vi "SDI Multi-Axis Simultaneous Start.vi"() -> ()   [LabVIEW 2014]
uses:
  <vilib>/Platform/TimedLoop/XDataNode/timing_clust.ctl
  <vilib>/Platform/TimedLoop/XDataNode/nitl_modes.ctl
  <vilib>/Platform/TimedLoop/XDataNode/wakeup.ctl
  <vilib>/Motion/plugins/PluginFramework/nismSDIFramework.SetFrameworkMode.multi.vi
  <vilib>/Motion/Express/_s/nimc.ex.clearFaults.clearFaults.axis.vi
  <vilib>/Motion/Express/_s/nimc.ex.power.power.axis.vi
  <vilib>/Motion/Express/_s/nimc.ex.read.readExecutionData.axis.vi
  <vilib>/Motion/Express/_s/nimc.ex.stopMove.stop.axis.modeDecelerate.vi
  <vilib>/Motion/Express/_s/nimc.ex.straightLineMove.startStraightLineMove.axis.modeRelative.0.vi
  <vilib>/Motion/BlockNode/FB.NIMotion.xnode
  <vilib>/Platform/TimedLoop/XDataNode/XDataNode.xnode
  <vilib>/Platform/TimedLoop/XDataNode/XDNodeRunTimeDep.lvlib
  <vilib>/Motion/plugins/SDI Plug-in - Delta ASDA/Template SoftMotion Drive Interface Plug-in Class.lvclass
panel:
  out "Move Done":bool
  out "Move Position":cluster{dbl, dbl}(graph)
  in  "Axis 2":refnum<k21>="Axis 2"
  in  "Velocity 2":dbl=3000.0
  in  "Position 2":dbl=7000.0
  in  "Stop Move":bool
  out "error out":errorcluster
  in  "Velocity 1":dbl=1000.0
  in  "Position 1":dbl=-4000.0
  out "Example Done":bool
  in  "Axis 1":refnum<k21>="Axis 1"
  # "Move Constraints"
  # "Notes: \n1. This example uses preconfigured settings that may not be appropriate for your motion system. Review and update the axis settings using the Axis Configuration dialog box. Right-click each axis and select Properties to open the Axis Configuration dialog box. \n2. Running this example automatically activates all axes. Disable the \"Enable Drive on Transition to Active Mode\" option on the General Settings page of the Axis Configuration dialog box to prevent axes from activating when the VI runs.\n3. This example uses the default smoothing input to automatically calculate deceleration and jerk values. To specify these move constraints, connect a control to the \"smoothing\" input to adjust the value to your requirements. \n\nFor information about using this example in an actual motion system, refer to ni.com/info and enter Info Code nismex."
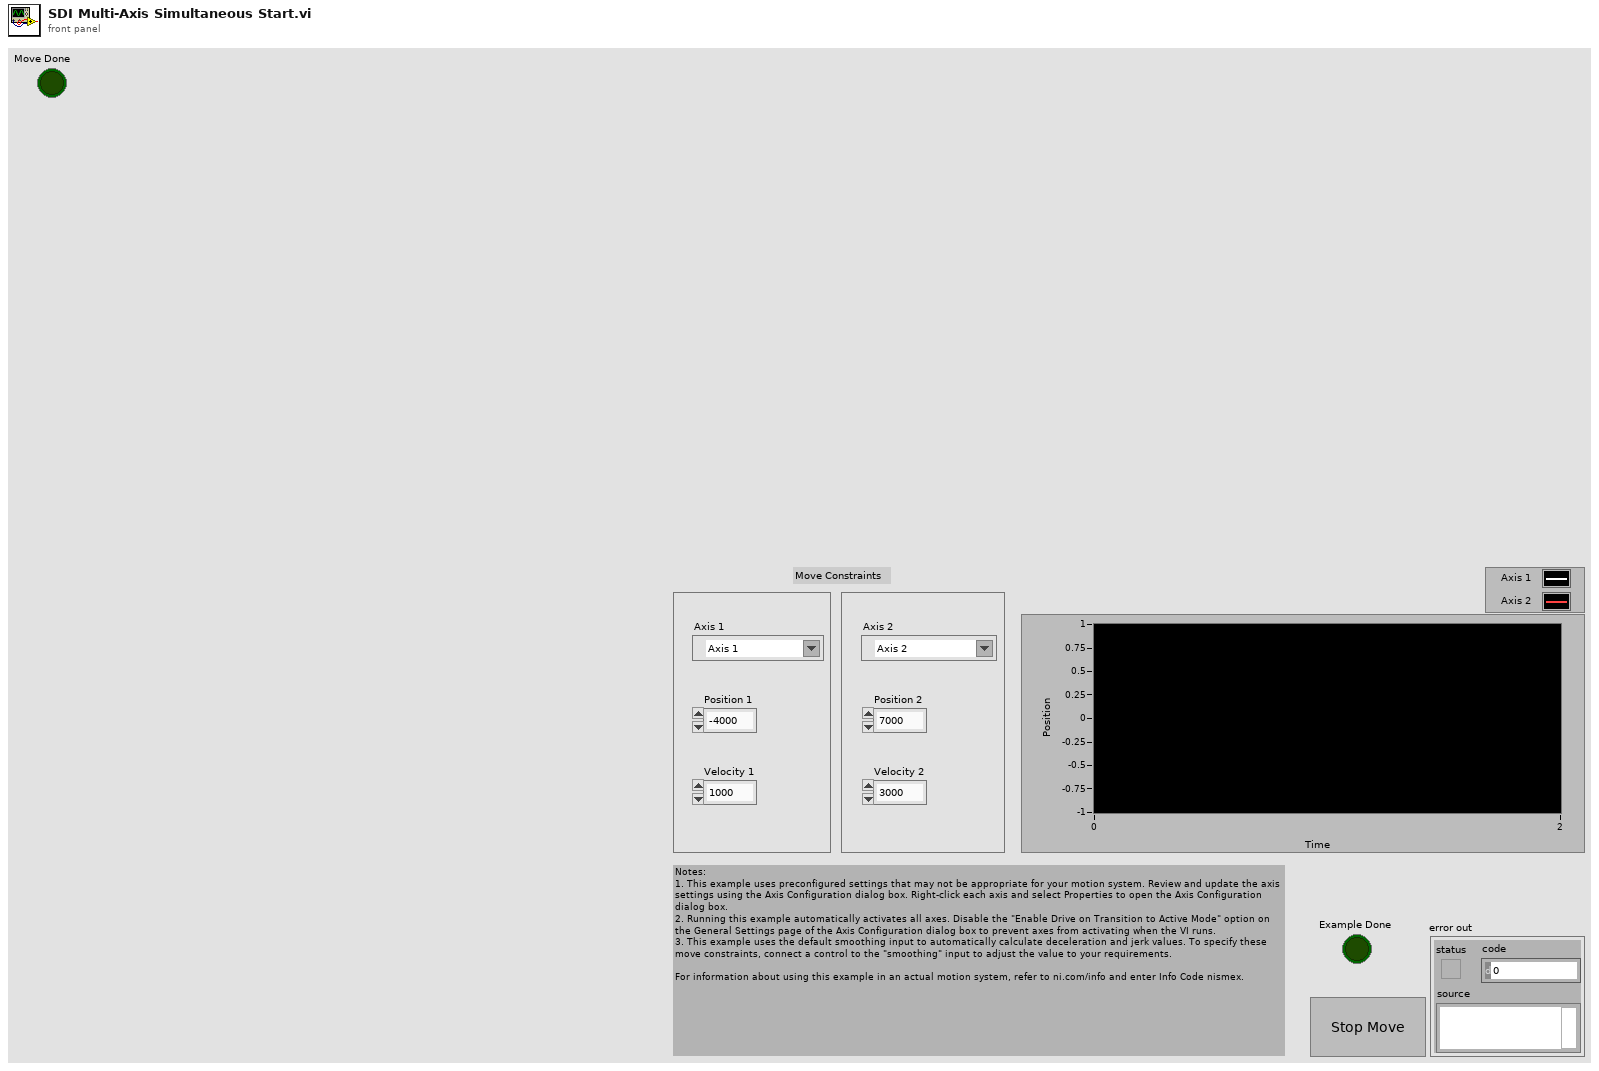
[diagram p1: front panel]
types:
  T1 = typedef "XDNodeRunTimeDep.lvlib/timing_clust.ctl" = cluster{"Expected End [f-1]":u64, "Actual End [f-1]":u64, "Finished Late? [f-1]":bool, "Expected End [i-1]":u64, "Actual End [i-1]":u64, "Finished Late? [i-1]":bool, "Expected Start [i]":u64, "Actual Start [i]":u64, "Expected Start [f]":u64, "Actual Start [f]":u64, "Source Name":string, "Structure Name":string, "Period":i64, "Deadline":i64, "Offset":i64, "Start":i64, "Priority":i32, "Timeout":i32, "Mode":T2, "Wakeup Reason":T3, "Error":errorcluster, "Source Type":string, "Secondary Source Type":string, "Global End Time":u64, "Global Start Time":u64, "Frame Duration":u64, "Iteration Duration":u64, "Assigned CPU":i32, "I/O Scan Engine Mode":u32}
  T2 = typedef "XDNodeRunTimeDep.lvlib/nitl_modes.ctl" = enum32{"No Change", "Process missed periods, maintain original phase", "Discard missed periods, maintain original phase", "Process missed periods, ignore original phase", "Discard missed periods, ignore original phase"}
  T3 = typedef "XDNodeRunTimeDep.lvlib/wakeup.ctl" = enum32{"Normal", "Aborted", "Asynchronous wakeup", "Timing source error", "Timed loop error", "Timeout"}
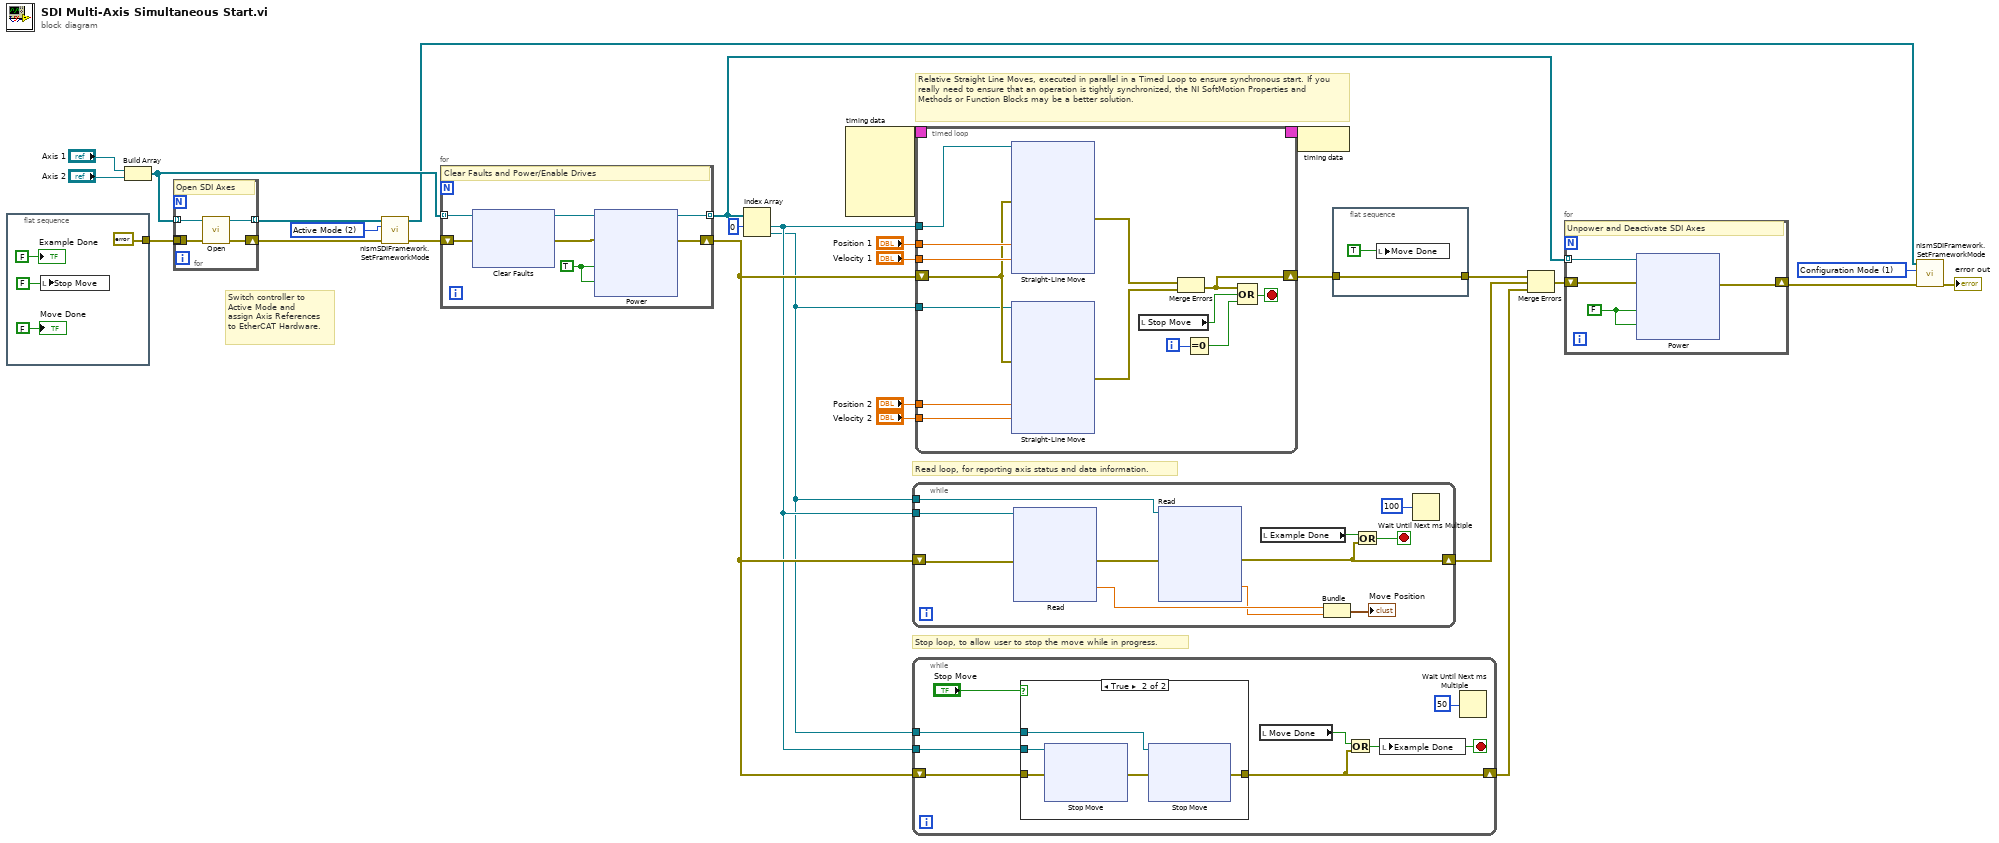
[diagram p0: block diagram]
diagram:
  w8 = 1 items=["Configuration Mode"=1, "Active Mode"=2] ("mode (Active Mode)")
  w18 = 2 items=["Configuration Mode"=1, "Active Mode"=2] ("mode (Active Mode)")
  # "Switch controller to\nActive Mode and \nassign Axis References\nto EtherCAT Hardware."
  # "Relative Straight Line Moves, executed in parallel in a Timed Loop to ensure synchronous start. If you really need to ensure that an operation is tightly synchronized, the NI SoftMotion Properties and Methods or Function Blocks may be a better solution."
  # "Read loop, for reporting axis status and data information."
  # "Stop loop, to allow user to stop the move while in progress."
  n1 = flat-sequence {
    tunnel: [w29] -> _
    tunnel: [w29] -> w11
    frame #0 {
      w29 = errorcluster {"status"=FALSE, "code"=0, "source"=""} ("Error")
      n2 = local write "Stop Move"(FALSE ("Example Done")) -> ()
      "Example Done" <- FALSE ("Example Done")
      "Move Done" <- FALSE ("Example Done")
    }
  }
  n3 = Build Array("Axis 1", "Axis 2") -> (w16:refnum<k21>[])
  n4 = for {
    tunnel: w16 -> [w36] mode=indexing
    tunnel: [w35] -> w15 mode=indexing
    shift-right: [w34] -> w14
    shift-left: _ -> [w33]
    tunnel: w11 -> [_]
    # "Open SDI Axes"
    n5 = call <vilib>:"Open.vi"("error in (no error)"=w33, "Axis"=w36) -> ("error out"=w34:errorcluster, "Base Axis Out"=w35:refnum<class "nismPluginAxisBaseClass.lvclass">)  [unwired: 8 in]
  }
  n6 = call-poly <vilib>:"nismSDIFramework.SetFrameworkMode.vi"("error in (no error)"=w14, "mode (Active Mode)"=w18, "Base Axis In"=w15) -> ("error out"=w17:errorcluster, "Base Axis Out"=w1:refnum<class "nismPluginAxisBaseClass.lvclass">[])  [unwired: 7 in]
  n7 = for {
    tunnel: w16 -> [w39] mode=indexing
    tunnel: [w38] -> w4 mode=indexing
    shift-right: [w41] -> w9
    shift-left: w17 -> [w40]
    w43 = TRUE ("enable axis")
    # "Clear Faults and Power/Enable Drives"
    n8 = xnode ("Clear Faults")("resource"=w39, "error in"=w40) -> ("resource out"=w37:refnum<k21>, "error out"=w42:errorcluster)
    n9 = xnode ("Power")("enable axis"=w43, "enable drive"=w43, "resource"=w37, "error in"=w42) -> ("resource out"=w38:refnum<k21>, "error out"=w41:errorcluster)
  }
  n10 = Index Array(array=w4, index #1=0 ("index")) -> (element #1=w3:refnum<k21>, element #2=w2:refnum<k21>)  [unwired: 1 in]
  n11 = node-c288() -> (w26:T1)  [unwired: 1 in, 4 out]
  n12 = while {
    shift-right: [w60] -> w28
    shift-left: w9 -> [w64]
    tunnel: w3 -> [w59]
    tunnel: w2 -> [w58]
    stop <- w67 stop-if-true
    n13 = xnode ("Read")("resource"=w59, "error in"=w64) -> ("position"=w68:dbl, "error out"=w62:errorcluster)  [unwired: 5 out]
    n14 = xnode ("Read")("resource"=w58, "error in"=w62) -> ("position"=w63:dbl, "error out"=w60:errorcluster)  [unwired: 5 out]
    n15 = local read "Example Done"() -> (w66:bool)
    n16 = Bundle("position"=w68, "position"=w63) -> (→"Move Position":cluster{"position":dbl, "position":dbl})  [unwired: 1 out]
    n17 = Or(x=w66, y=w60) -> (x .or. y?=w67:bool)
    n18 = Wait Until Next ms Multiple(millisecond multiple=u32 100) -> ()  [unwired: 1 out]
  }
  n19 = while {
    shift-right: [w90] -> w27
    shift-left: w9 -> [w92]
    tunnel: w3 -> [w88]
    tunnel: w2 -> [w87]
    stop <- w89 stop-if-true
    n20 = case shown="True" "Stop Move" {
      tunnel: [w95 w100] -> w90
      tunnel: w92 -> [w95 w99]
      tunnel: w88 -> [_ w97]
      tunnel: w87 -> [_ w96]
      frame False {
      }
      frame True {
        n21 = xnode ("Stop Move")("resource"=w97, "error in"=w99) -> ("error out"=w98:errorcluster)  [unwired: 1 in, 2 out]
        n22 = xnode ("Stop Move")("resource"=w96, "error in"=w98) -> ("error out"=w100:errorcluster)  [unwired: 1 in, 2 out]
      }
    }
    n23 = local read "Move Done"() -> (w91:bool)
    n24 = Or(x=w91, y=w90) -> (x .or. y?=w89:bool)
    n25 = local write "Example Done"(w89) -> ()
    n26 = Wait Until Next ms Multiple(millisecond multiple=u32 50) -> ()  [unwired: 1 out]
  }
  n27 = timed-loop {
    timing: w26 -> [_]
    timing-out: [_] -> w25
    tunnel: "Position 2" -> [w130]
    tunnel: "Velocity 2" -> [w129]
    tunnel: "Position 1" -> [w128]
    tunnel: "Velocity 1" -> [w127]
    shift-right: [w122] -> w19
    shift-left: w9 -> [w123]
    tunnel: w3 -> [w118]
    tunnel: w2 -> [w117]
    i -> [w119]
    stop <- w126 stop-if-true
    n28 = xnode ("Straight-Line Move")("position"=w128, "velocity"=w127, "resource"=w118, "error in"=w123) -> ("error out"=w124:errorcluster)  [unwired: 6 in, 2 out]
    n29 = xnode ("Straight-Line Move")("position"=w130, "velocity"=w129, "resource"=w117, "error in"=w123) -> ("error out"=w125:errorcluster)  [unwired: 6 in, 2 out]
    n30 = local read "Stop Move"() -> (w121:bool)
    n31 = Merge Errors(w124, w125) -> (w122:errorcluster)
    n32 = Equal To 0?(x=w119) -> (x = 0?=w120:bool)
    n33 = Compound Arithmetic op=OR(w122, w121, w120) -> (w126:bool)
  }
  n34 = node-c288(w25) -> ()
  n35 = flat-sequence {
    tunnel: w19 -> [w163]
    tunnel: [w163] -> w20
    frame #0 {
      n36 = local write "Move Done"(TRUE ("Example Done")) -> ()
    }
  }
  n37 = Merge Errors(w20, w28, w27) -> (w6:errorcluster)
  n38 = for {
    tunnel: w4 -> [w165] mode=indexing
    shift-right: [w167] -> w7
    shift-left: w6 -> [w166]
    w168 = FALSE ("enable axis")
    # "Unpower and Deactivate SDI Axes"
    n39 = xnode ("Power")("enable axis"=w168, "enable drive"=w168, "resource"=w165, "error in"=w166) -> ("error out"=w167:errorcluster)  [unwired: 1 out]
  }
  n40 = call-poly <vilib>:"nismSDIFramework.SetFrameworkMode.vi"("error in (no error)"=w7, "mode (Active Mode)"=w8, "Base Axis In"=w1) -> ("error out"=→"error out":errorcluster)  [unwired: 7 in, 1 out]
